vi "Read Aalborg GFC17 Connections.vi"(8 "error in (no error)":errorcluster, 11 "Aalborg GFC17 in":refnum<class "Aalborg GFC17.lvclass">) -> (0 "error out":errorcluster, 2 "Aalborg GFC17 Connections":T1={"flow rate setpoint channel"="cDAQ1Mod3/ao0", "flow rate reading channel"="cDAQ1Mod1/ai4", "valve channel"="cDAQ1Mod3/ao1"}, 3 "Aalborg GFC17 out":refnum<class "Aalborg GFC17.lvclass">)   [LabVIEW 2011, in "Aalborg GFC17.lvclass"]
uses:
  Aalborg GFC17.lvclass
  Aalborg GFC17 Connections.ctl
  Aalborg GFC17.lvclass/Aalborg GFC17.ctl
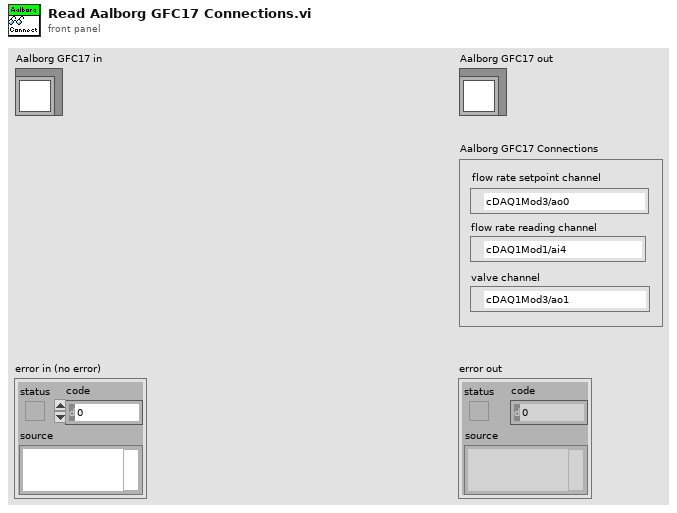
[diagram p1: front panel]
types:
  T1 = typedef "Aalborg GFC17.lvclass/Aalborg GFC17 Connections.ctl" = cluster{"flow rate setpoint channel":tag, "flow rate reading channel":tag, "valve channel":tag}
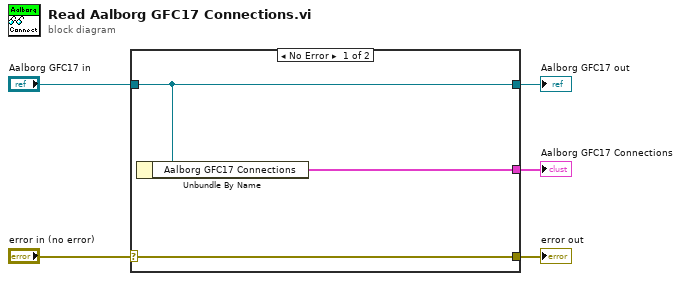
[diagram p0: block diagram]
diagram:
  n1 = case shown="No Error" "error in (no error)" {
    selector: "error in (no error)" -> [w8 w9]
    tunnel: [w8 w9] -> w4
    tunnel: [w7 w10] -> w2
    tunnel: "Aalborg GFC17 in" -> [w7 w10]
    tunnel: [w6 _] -> w1
    frame No Error {
      n2 = Unbundle By Name(w7) -> ("Aalborg GFC17 Connections"=w6:T1)
    }
    frame Error {
    }
  }
  "error out" <- w4
  "Aalborg GFC17 out" <- w2
  "Aalborg GFC17 Connections" <- w1
